vi "Écrire_n_splits.vi"(8 "error in (no error)":errorcluster caption="entrée d'erreur (pas d'erreur)", 10 "n_splits":u8, 11 "Splitter en entrée":refnum<class "Splitter.lvclass">) -> (0 "error out":errorcluster caption="sortie d'erreur", 3 "Splitter en sortie":refnum<class "Splitter.lvclass">)   [LabVIEW 2020, in "Splitter.lvclass"]
uses:
  Splitter.lvclass
  Splitter.lvclass/Splitter.ctl
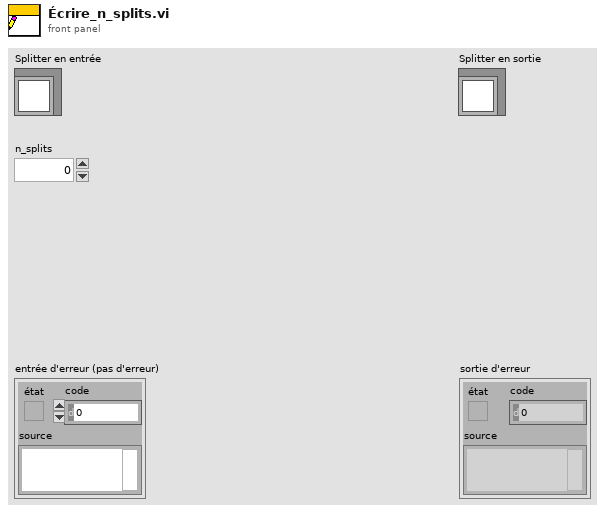
[diagram p1: front panel]
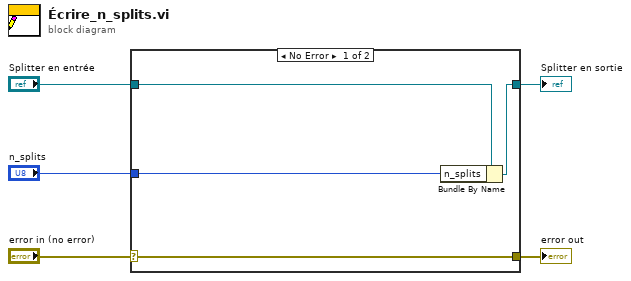
[diagram p0: block diagram]
diagram:
  n1 = case shown="No Error" "error in (no error)" {
    selector: "error in (no error)" -> [w9 w10]
    tunnel: [w9 w10] -> w4
    tunnel: [w7 w11] -> w2
    tunnel: "Splitter en entrée" -> [w8 w11]
    tunnel: "n_splits" -> [w6 _]
    frame No Error {
      n2 = Bundle By Name(cluster=w8, "n_splits"=w6) -> (w7:refnum<class "Splitter.lvclass">)
    }
    frame Error {
    }
  }
  "error out" <- w4
  "Splitter en sortie" <- w2
